vi "BaseProvider_ActorFramework_FindTemplates.vi"(9 "MainClassemplateID":string, 10 "FilterOnProviders":string, 11 "DeriveFromClassRef":refnum<vi>) -> (2 "ActorsTemplatesFound":bool, 3 "Array":T1[](array[typedef]))   [LabVIEW 2020]
uses:
  <resource>/Framework/Providers/Open_GDS/ClassProviders/Provider_BaseClassInterface/ClassTemplateType.ctl
  <vilib>/Utility/config.llb/Read Key (String).vi
  <resource>/Framework/Providers/Open_GDS/ClassProviders/Provider_BaseClassInterface/ClassWriter_class/ClassWriter.lvclass
  <vilib>/Utility/config.llb/NI_LVConfig.lvlib
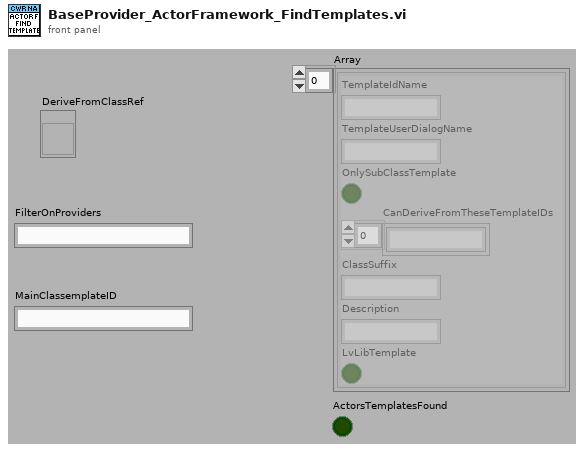
[diagram p1: front panel]
types:
  T1 = typedef "ClassWriter.lvclass/ClassTemplateType.ctl" = cluster{"TemplateIdName":string, "TemplateUserDialogName":string, "OnlySubClassTemplate":bool, "CanDeriveFromTheseTemplateIDs":string[], "ClassSuffix":string, "Description":string, "LvLibTemplate":bool}
  T2 = typedef "NI_LVConfig.lvlib/Config Data RefNum.ctl" = refnum<k1>
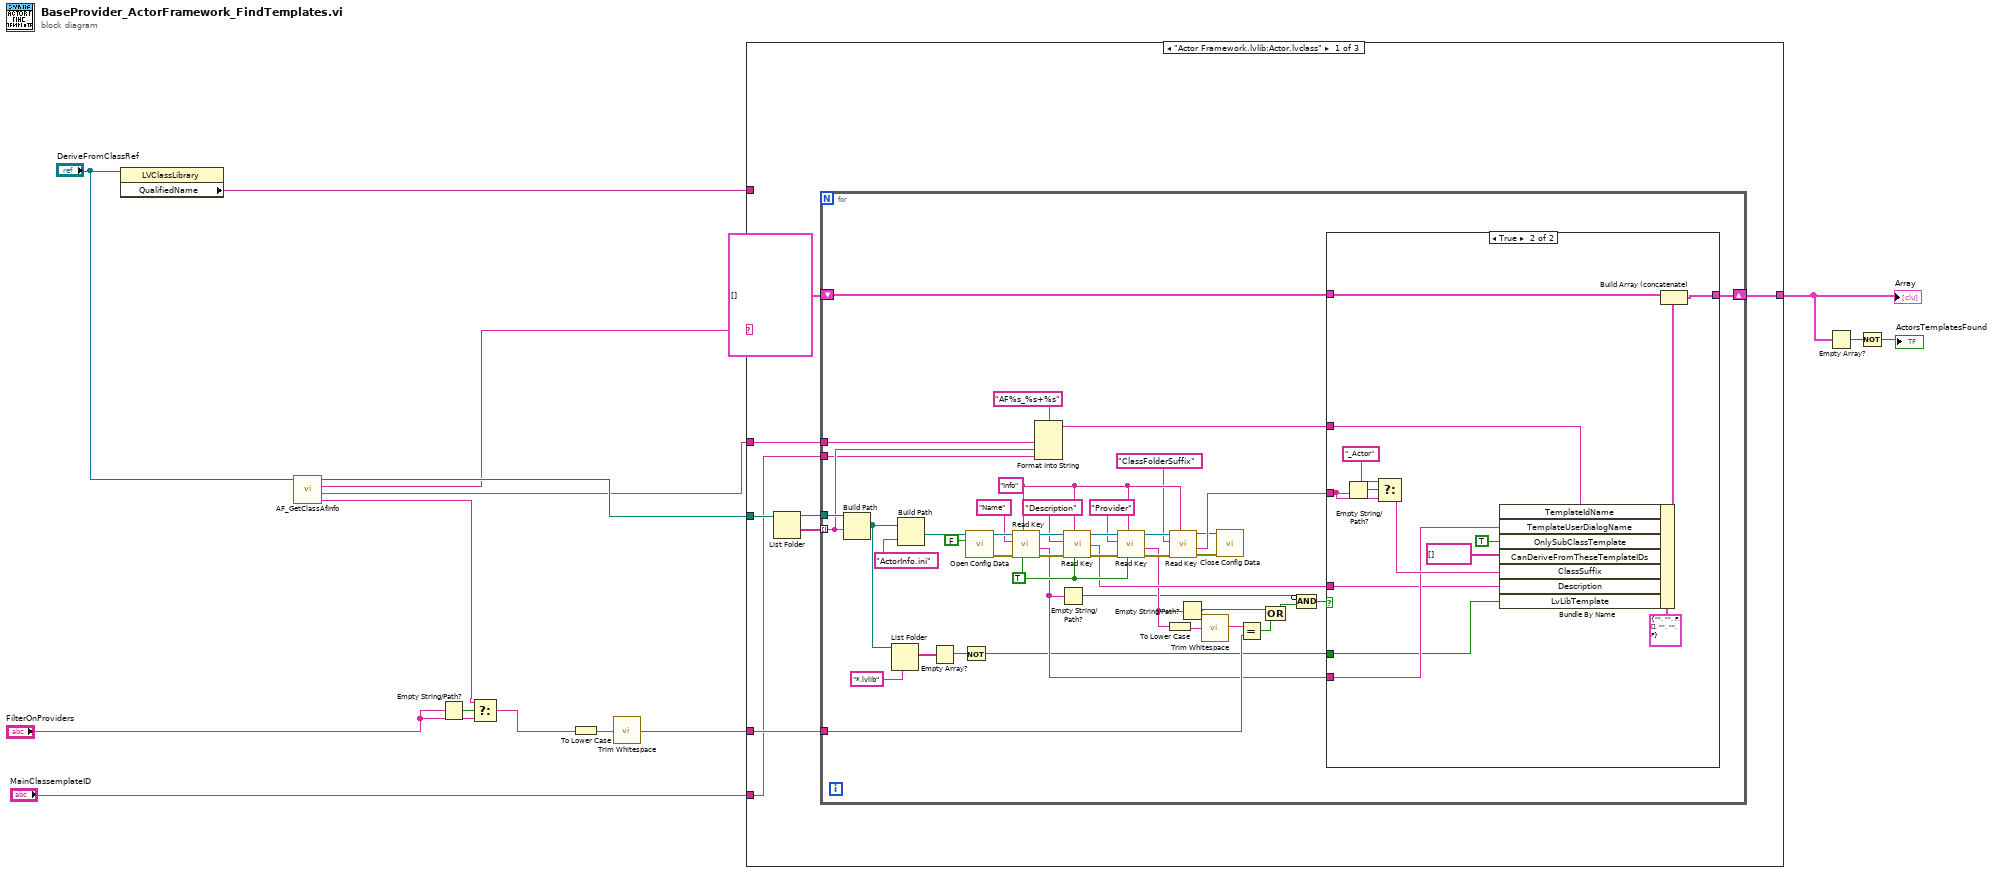
[diagram p0: block diagram]
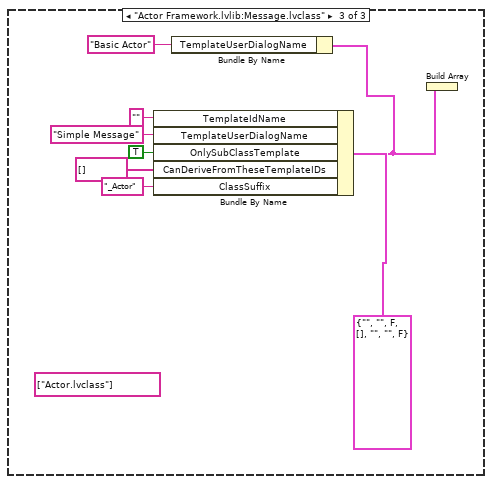
[diagram p4: hidden frame]
diagram:
  n1 = property class="LVClassLibrary"(reference="DeriveFromClassRef") -> ("QualifiedName"=w15:string)  [unwired: 1 in, 2 out]
  n2 = call <resource>:"AF_GetClassAfInfo.vi"("DeriveFromClassRef"="DeriveFromClassRef") -> ("ClassSuffix"=w6:string, "TemplateIdName"=w12:string, "RootClassQualifiedName"=w1:string, "AF Folder Path"=w13:path)  [unwired: 5 in, 2 out]
  n3 = Empty String/Path?(string/path="FilterOnProviders") -> (empty?=w5:bool)
  n4 = Select(t=w6, s=w5, f="FilterOnProviders") -> (s? t:f=w3:string)
  n5 = To Lower Case(string=w3) -> (all lower case string=w11:string)
  n6 = call <vilib>:"Trim Whitespace.vi"("string"=w11) -> ("trimmed string"=w10:string)  [unwired: 1 in]
  n7 = case shown="\"Actor Framework.lvlib:Actor.lvclass\"" w1 {
    tunnel: w15 -> [_ _ _]
    tunnel: w13 -> [w23 _ _]
    tunnel: w12 -> [w20 _ _]
    tunnel: w10 -> [w19 _ _]
    tunnel: [w18 _ _] -> w9
    tunnel: "MainClassemplateID" -> [w16 _ _]
    frame "Actor Framework.lvlib:Actor.lvclass" {
      n8 = List Folder(path=w23) -> (path out=w21:path, folder names=w22:string[])  [unwired: 3 in, 2 out]
      n9 = for {
        tunnel: w22 -> [w63] mode=indexing
        tunnel: w21 -> [w67]
        tunnel: w20 -> [w64]
        tunnel: w19 -> [w49]
        shift-right: [w42] -> w18
        shift-left: T1[] [] -> [w43]
        tunnel: w16 -> [w24]
        w45 = "Info" ("section")
        w61 = TRUE ("read raw string? (F)")
        n10 = Build Path(base path=w67, name or relative path=w63) -> (appended path=w29:path)
        n11 = List Folder(path=w29, pattern="*.lvlib") -> (filenames=w27:string[])  [unwired: 2 in, 3 out]
        n12 = Build Path(base path=w29, name or relative path="ActorInfo.ini") -> (appended path=w54:path)
        n13 = Empty Array?(array=w27) -> (empty?=w26:bool)
        n14 = Not(x=w26) -> (.not. x?=w25:bool)
        n15 = call <vilib>:"Open Config Data.vi"("create file if necessary (T)"=FALSE, "configuration file path"=w54) -> ("error out"=w55:errorcluster, "refnum"=w56:T2)  [unwired: 7 in, 1 out]
        n16 = call-poly <vilib>:"Read Key.vi"("read raw string? (F)"=w61, "section"=w45, "error in (no error)"=w55, "key"="Name", "refnum"=w56) -> ("error out"=w58:errorcluster, "value"=w35:string, "refnum out"=w57:T2)  [unwired: 3 in, 1 out]
        n17 = Format Into String(format string="AF%s_%s+%s", w64, w63, w24) -> (resulting string=w62:string)  [unwired: 2 in, 1 out]
        n18 = Empty String/Path?(string/path=w35) -> (empty?=w32:bool)
        n19 = call-poly <vilib>:"Read Key.vi"("read raw string? (F)"=w61, "section"=w45, "error in (no error)"=w58, "key"="Description", "refnum"=w57) -> ("error out"=w60:errorcluster, "value"=w40:string, "refnum out"=w59:T2)  [unwired: 3 in, 1 out]
        n20 = call-poly <vilib>:"Read Key.vi"("read raw string? (F)"=w61, "section"=w45, "error in (no error)"=w60, "key"="Provider", "refnum"=w59) -> ("error out"=w47:errorcluster, "value"=w38:string, "refnum out"=w48:T2)  [unwired: 3 in, 1 out]
        n21 = To Lower Case(string=w38) -> (all lower case string=w39:string)
        n22 = call-poly <vilib>:"Read Key.vi"("section"=w45, "error in (no error)"=w47, "key"="ClassFolderSuffix", "refnum"=w48) -> ("error out"=w37:errorcluster, "value"=w41:string, "refnum out"=w36:T2)  [unwired: 4 in, 1 out]
        n23 = Empty String/Path?(string/path=w38) -> (empty?=w33:bool)
        n24 = call <vilib>:"Trim Whitespace.vi"("string"=w39) -> ("trimmed string"=w50:string)  [unwired: 1 in]
        n25 = call <vilib>:"Close Config Data.vi"("error in (no error)"=w37, "refnum"=w36) -> ()  [unwired: 8 in, 2 out]
        n26 = Equal?(x=w50, y=w49) -> (x = y?=w34:bool)
        n27 = Compound Arithmetic op=OR(w33, w34) -> (w31:bool)
        n28 = Compound Arithmetic op=AND(invert w32, w31) -> (w30:bool)
        n29 = case shown="True" w30 {
          tunnel: w62 -> [_ w79]
          tunnel: w43 -> [w68 w78]
          tunnel: [w68 w76] -> w42
          tunnel: w41 -> [_ w73]
          tunnel: w35 -> [_ w71]
          tunnel: w40 -> [_ w70]
          tunnel: w25 -> [_ w69]
          frame False {
          }
          frame True {
            n30 = Empty String/Path?(string/path=w73) -> (empty?=w75:bool)
            n31 = Select(t="_Actor" ("ClassSuffix"), s=w75, f=w73) -> (s? t:f=w72:string)
            n32 = Bundle By Name(cluster=T1 {"TemplateIdName"="", "TemplateUserDialogName"="", "OnlySubClassTemplate"=FALSE, "CanDeriveFromTheseTemplateIDs"=[], "ClassSuffix"="", "Description"="", "LvLibTemplate"=FALSE} ("ClassTemplateType"), "TemplateIdName"=w79, "TemplateUserDialogName"=w71, "OnlySubClassTemplate"=TRUE, "CanDeriveFromTheseTemplateIDs"=string[] [], "ClassSuffix"=w72, "Description"=w70, "LvLibTemplate"=w69) -> (w77:T1)
            n33 = Build Array (concatenate)(w78, w77) -> (w76:T1[])
          }
        }
      }
    }
    frame Default {
    }
    frame "Actor Framework.lvlib:Message.lvclass" {
      (unwired) string[] ["Actor.lvclass"] ("CanDeriveFromTheseTemplateIDs")
      n34 = Bundle By Name(cluster=T1 {"TemplateIdName"="", "TemplateUserDialogName"="", "OnlySubClassTemplate"=FALSE, "CanDeriveFromTheseTemplateIDs"=[], "ClassSuffix"="", "Description"="", "LvLibTemplate"=FALSE} ("ClassTemplateType"), "TemplateIdName"="", "TemplateUserDialogName"="Simple Message", "OnlySubClassTemplate"=TRUE, "CanDeriveFromTheseTemplateIDs"=string[] [], "ClassSuffix"="_Actor") -> (w86:T1)
      n35 = Bundle By Name(cluster=w86, "TemplateUserDialogName"="Basic Actor") -> ()  [unwired: 1 out]
      n36 = Build Array(w86) -> ()  [unwired: 1 out]
    }
  }
  "Array" <- w9
  n37 = Empty Array?(array=w9) -> (empty?=w8:bool)
  n38 = Not(x=w8) -> (.not. x?=→"ActorsTemplatesFound":bool)
